vi "WFLastSampleToBaselineA.vi"(4 "error in (no error)":errorcluster, 6 "Baseline":dbl, 7 "Waveform In":waveform(dbl)={"t0"=timestamp(0 s since 1904-01-01), "dt"=0.0, "Y"=[]}) -> (0 "error out":errorcluster, 3 "Waveform Out":waveform(dbl))   [LabVIEW 2013]
doc: "Makes sure that last sample of waveform is at baseline. This is important if streaming this waveform to a DAQ card."
uses:
  <vilib>/Waveform/WDTOps.llb/WDT Number of Waveform Samples DBL.vi
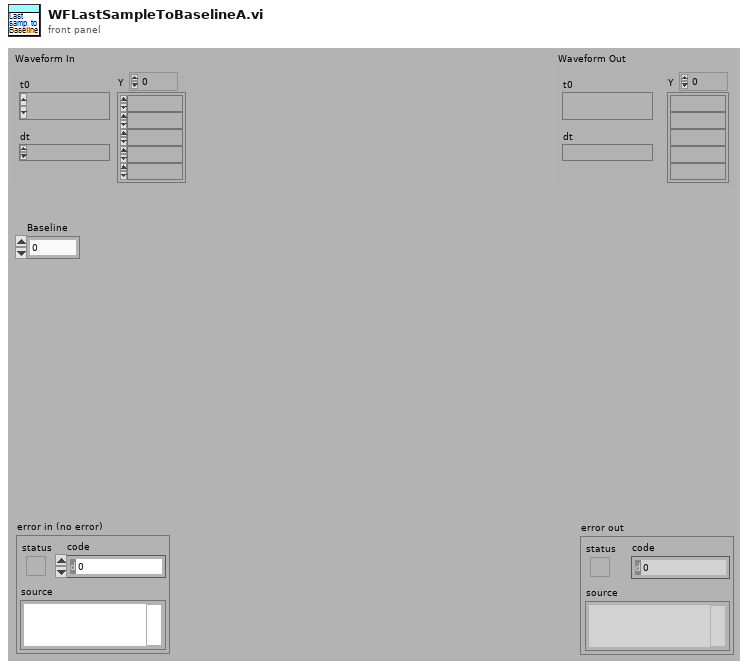
[diagram p1: front panel]
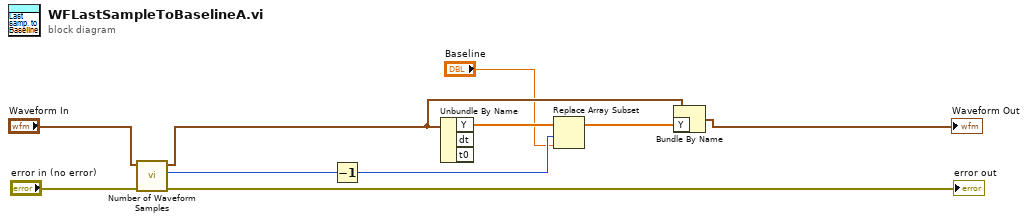
[diagram p0: block diagram]
diagram:
  n1 = call-poly <vilib>:"Number of Waveform Samples.vi"("error in (no error)"="error in (no error)", "waveform in"="Waveform In") -> ("error out"=→"error out":errorcluster, "number of samples"=w3:i32, "waveform out"=w7:waveform(dbl))  [unwired: 7 in]
  n2 = Decrement(x=w3) -> (x-1=w2:i32)
  n3 = Unbundle By Name(w7) -> ("Y"=w5:dbl[])  [unwired: 2 out]
  n4 = Replace Array Subset(array=w5, new element="Baseline", index=w2) -> (w4:dbl[])
  n5 = Bundle By Name(cluster=w7, "Y"=w4) -> (→"Waveform Out":waveform(dbl))
